vi "FTW-JSON-Object-GetElement-Bool.vi"(0 "JSON":refnum<class "FTW-Container.lvclass">, 5 "Key":string, 7 "Default Value":bool, 9 "Remove Value":bool, 11 "error in":errorcluster) -> (4 "JSON out":refnum<class "FTW-Container.lvclass">, 6 "JSON Element Type":T1, 8 "Value":bool, 15 "error out":errorcluster)   [LabVIEW 2015]
uses:
  container/FTW-Container.lvclass
  FTW-JSON-Type.ctl
panel:
  # "Inputs"
  # "Outputs"
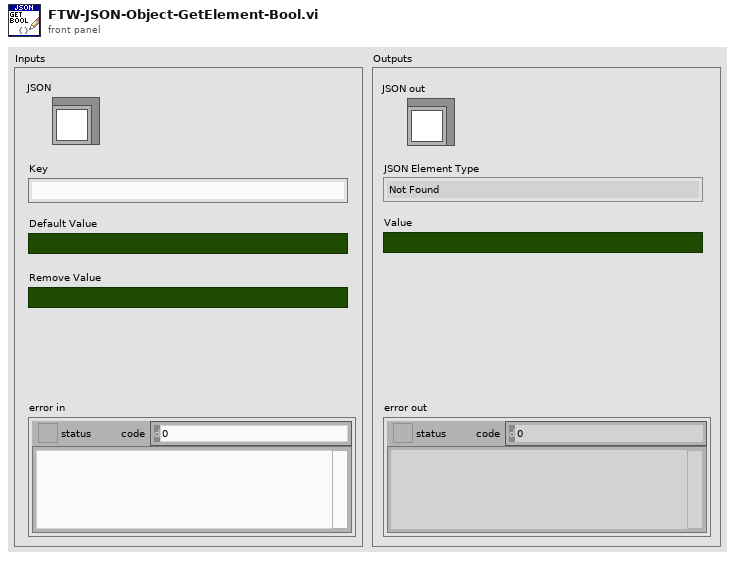
[diagram p1: front panel]
types:
  T1 = typedef "FTW-JSON-Type.ctl" = enum8{"Not Found", "Object", "Array", "String", "Number", "Boolean", "null"}
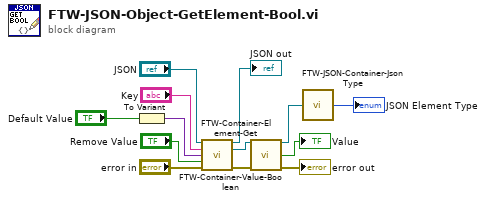
[diagram p0: block diagram]
diagram:
  n1 = To Variant(anything="Default Value") -> (Variant=w6:variant)
  n2 = call "FTW-Container-Element-Get.vi"("FTW-Container In"="JSON", "Element Name"="Key", "Default Value"=w6, "Delete?"="Remove Value", "error in"="error in") -> ("FTW-Container Out"=→"JSON out":refnum<class "FTW-Container.lvclass">, "Element Out"=w5:refnum<class "FTW-Container.lvclass">, "error out"=w12:errorcluster)  [unwired: 7 in, 1 out]
  n3 = call "FTW-Container-Value-Boolean.vi"("FTW-Container In"=w5, "error in"=w12) -> ("FTW-Container Out"=w1:refnum<class "FTW-Container.lvclass">, "Value"=→"Value":bool, "error out"=→"error out":errorcluster)  [unwired: 11 in]
  n4 = call "FTW-JSON-Container-JsonType.vi"("Container"=w1) -> ("JSON Element Type"=→"JSON Element Type":T1)  [unwired: 14 in]
